vi "GUNSC_GetImageGeom.vi"(11 "Database RefNum":T1) -> (1 "name":string, 2 "image struct":T2)   [LabVIEW 2016]
uses:
  DBSHAND/private/vis/DatabaseHand_RefNum.ctl
  DBSHAND/private/vis/DatabaseHand_Element_Get(bool).vi
  DBSHAND/private/vis/DatabaseHand_Element_Get(I32).vi
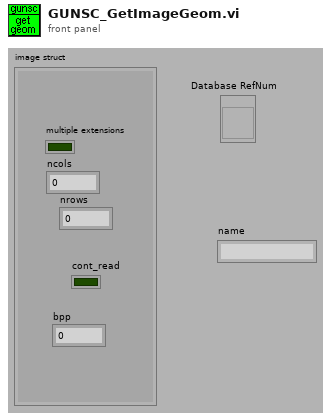
[diagram p1: front panel]
types:
  T1 = typedef "DatabaseHand_RefNum.ctl" = refnum<vi>
  T2 = cluster{"multiple extensions":bool, "ncols":u16, "nrows":u16, "bpp":i16, "cont_read":bool}
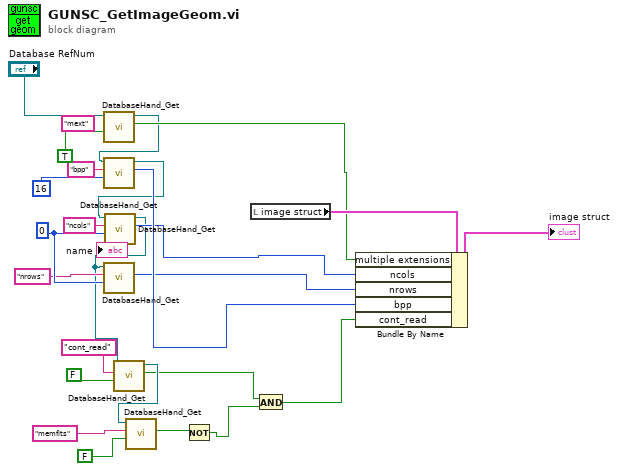
[diagram p0: block diagram]
diagram:
  w14 = 0
  (unwired) "mext" ("name")
  n1 = call-poly "DatabaseHand_Get.vi"("default value"=TRUE, "Database RefNum in"="Database RefNum") -> ("value"=w21:bool, "Database RefNum out"=w20:T1)  [unwired: 3 in, 5 out]
  n2 = call-poly "DatabaseHand_Get.vi"("default value"=16, "name"="bpp", "Database RefNum in"=w20) -> ("value"=w17:i32, "Database RefNum out"=w16:T1)  [unwired: 2 in, 5 out]
  n3 = call-poly "DatabaseHand_Get.vi"("default value"=w14, "name"="ncols", "Database RefNum in"=w16) -> ("value"=w11:i32, "Database RefNum out"=w9:T1)  [unwired: 2 in, 5 out]
  n4 = call-poly "DatabaseHand_Get.vi"("default value"=w14, "name"="nrows", "Database RefNum in"=w9) -> ("value"=w12:i32)  [unwired: 2 in, 6 out]
  n5 = call-poly "DatabaseHand_Get.vi"("default value"=FALSE, "name"="cont_read", "Database RefNum in"=w9) -> ("value"=w2:bool, "Database RefNum out"=w6:T1)  [unwired: 2 in, 5 out]
  n6 = call-poly "DatabaseHand_Get.vi"("default value"=FALSE, "name"="memfits", "Database RefNum in"=w6) -> ("value"=w4:bool)  [unwired: 2 in, 6 out]
  n7 = Not(x=w4) -> (.not. x?=w3:bool)
  n8 = local read "image struct"() -> (w25:T2)
  n9 = And(x=w2, y=w3) -> (x .and. y?=w1:bool)
  n10 = Bundle By Name(cluster=w25, "multiple extensions"=w21, "ncols"=w11, "nrows"=w12, "bpp"=w17, "cont_read"=w1) -> (→"image struct":T2)
